vi "TransGen_mono (SubVI).vi"(6 "tau1":dbl step=0.1, 7 "A1":dbl step=100.0, 9 "step":dbl[](array[numeric]), 10 "time":dbl[](array[numeric]), 11 "Z":dbl) -> (3 "intensity":dbl[](array[numeric]))   [LabVIEW 2017]
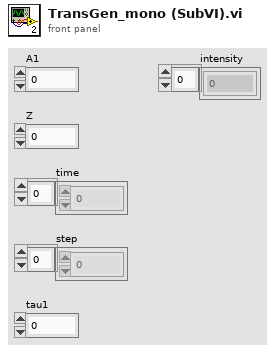
[diagram p1: front panel]
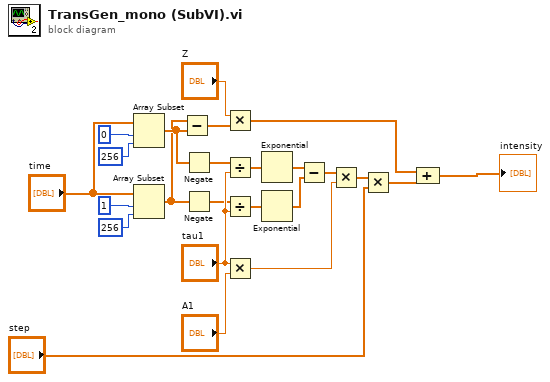
[diagram p0: block diagram]
diagram:
  n1 = Array Subset(array="time", index=0, length=256) -> (w19:dbl[])
  n2 = Array Subset(array="time", index=1, length=256) -> (w18:dbl[])
  n3 = Subtract(x=w18, y=w19) -> (x-y=w20:dbl[])
  n4 = Negate(x=w19) -> (-x=w2:dbl[])
  n5 = Negate(x=w18) -> (-x=w9:dbl[])
  n6 = Multiply(x="Z", y=w20) -> (x*y=w13:dbl[])
  n7 = Divide(x=w2, y="tau1") -> (x/y=w3:dbl[])
  n8 = Divide(x=w9, y="tau1") -> (x/y=w10:dbl[])
  n9 = Multiply(x="tau1", y="A1") -> (x*y=w16:dbl)
  n10 = Exponential(1:w3) -> (0:w11:dbl[])
  n11 = Exponential(1:w10) -> (0:w12:dbl[])
  n12 = Subtract(x=w11, y=w12) -> (x-y=w17:dbl[])
  n13 = Multiply(x=w17, y=w16) -> (x*y=w23:dbl[])
  n14 = Multiply(x=w23, y="step") -> (x*y=w22:dbl[])
  n15 = Compound Arithmetic op=ADD(w13, w22) -> (→"intensity":dbl[])
